vi "16_1.vi"() -> ()   [LabVIEW 2018]
panel:
  out "sum":i32
  out "your ticket":string
  out "nearby tickets":string[](array[string])
  out "first subarray":string[](array[string])
  in  "Input":string
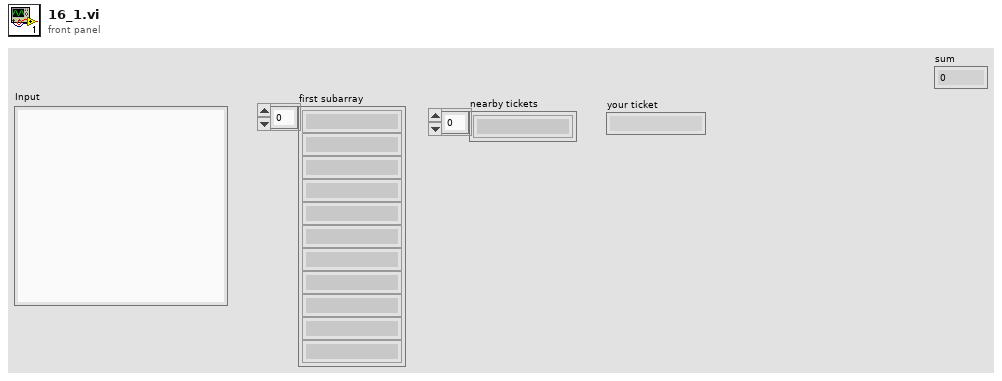
[diagram p1: front panel]
types:
  T1 = cluster{"Min1":i32, "Max1":i32, "Min2":i32, "Max2":i32}
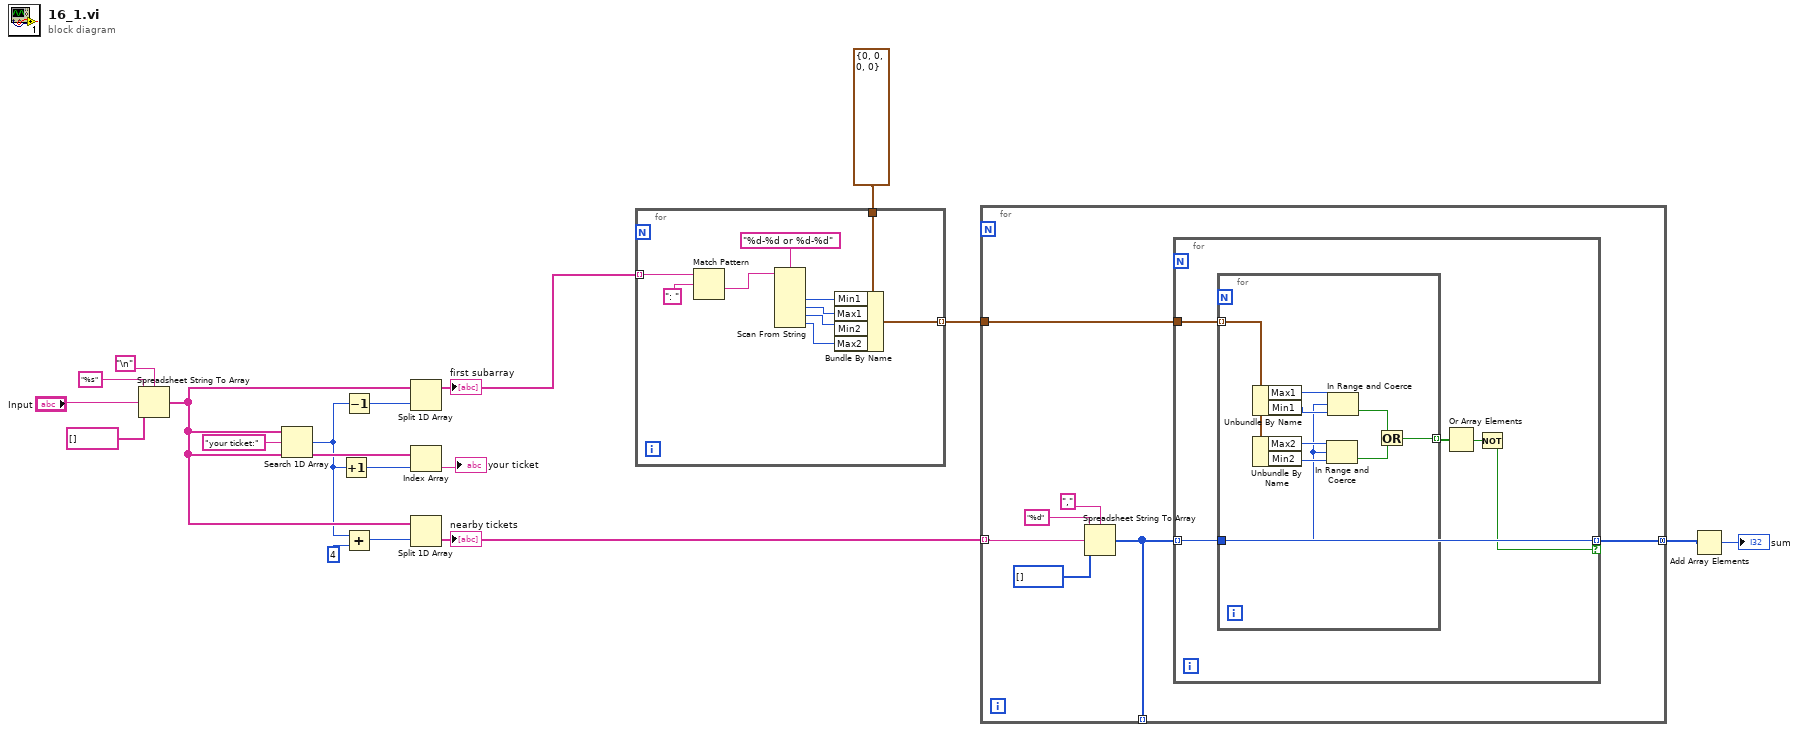
[diagram p0: block diagram]
diagram:
  n1 = Spreadsheet String To Array(delimiter (Tab)="\n", format string="%s", spreadsheet string="Input", array type (2D Dbl)=string[] []) -> (array=w11:string[])
  n2 = Search 1D Array(1D array=w11, element="your ticket:") -> (index of element=w9:i32)  [unwired: 1 in]
  n3 = Increment(x=w9) -> (x+1=w12:i32)
  n4 = Decrement(x=w9) -> (x-1=w13:i32)
  n5 = Add(x=w9, y=4) -> (x+y=w10:i32)
  n6 = Split 1D Array(array=w11, index=w13) -> (first subarray=w6:string[])  [unwired: 1 out]
  "first subarray" <- w6
  n7 = Index Array(array=w11, index=w12) -> (element=→"your ticket":string)
  n8 = Split 1D Array(array=w11, index=w10) -> (second subarray=w4:string[])  [unwired: 1 out]
  "nearby tickets" <- w4
  n9 = for {
    tunnel: w6 -> [w28] mode=indexing
    tunnel: T1 {"Min1"=0, "Max1"=0, "Min2"=0, "Max2"=0} -> [w24]
    tunnel: [w19] -> w3 mode=indexing
    n10 = Match Pattern(string=w28, regular expression=": ") -> (after substring=w26:string)  [unwired: 1 in, 3 out]
    n11 = Scan From String(format string="%d-%d or %d-%d", input string=w26) -> (output 1=w23:i32, output 2=w22:i32, output 3=w21:i32, output 4=w20:i32)  [unwired: 6 in, 3 out]
    n12 = Bundle By Name(cluster=w24, "Min1"=w23, "Max1"=w22, "Min2"=w21, "Max2"=w20) -> (w19:T1)
  }
  n13 = for {
    tunnel: w4 -> [w32] mode=indexing
    tunnel: w3 -> [w31]
    tunnel: [w30] -> w2 mode=concatenating
    tunnel: [w29] -> _ mode=indexing
    n14 = Spreadsheet String To Array(delimiter (Tab)=",", format string="%d", spreadsheet string=w32, array type (2D Dbl)=i32[] []) -> (array=w29:i32[])
    n15 = for {
      tunnel: w29 -> [w37] mode=indexing
      tunnel: w31 -> [w40]
      tunnel: [w37] -> w30 mode=indexing if=w36
      n16 = for {
        tunnel: w40 -> [w45] mode=indexing
        tunnel: w37 -> [w42]
        tunnel: [w41] -> w39 mode=indexing
        n17 = Unbundle By Name(w45) -> ("Max1"=w49:i32, "Min1"=w48:i32)
        n18 = Unbundle By Name(w45) -> ("Max2"=w47:i32, "Min2"=w46:i32)
        n19 = In Range and Coerce(upper limit=w47, x=w42, lower limit=w46) -> (In Range?=w44:bool)  [unwired: 1 out]
        n20 = In Range and Coerce(upper limit=w49, x=w42, lower limit=w48) -> (In Range?=w43:bool)  [unwired: 1 out]
        n21 = Or(x=w43, y=w44) -> (x .or. y?=w41:bool)
      }
      n22 = Or Array Elements(Boolean array=w39) -> (logical OR=w38:bool)
      n23 = Not(x=w38) -> (.not. x?=w36:bool)
    }
  }
  n24 = Add Array Elements(numeric array=w2) -> (sum=→"sum":i32)
